vi "SolveContinousARE.vi"(8 "R":T3=[[1.0]], 9 "Q":T3=[[10.0, 0.0], [0.0, 100.0]], 10 "B":T3=[[0.0], [1.0]], 11 "A":T3=[[0.0, 1.0], [0.0, -1.0]]) -> (3 "A x B":T1=[[-1.6028844918025698e-15+0.0i, -100.90089284923441+0.0i], [-0.09910715076567198+0.0i, -1.0000000000000013+0.0i]])   [LabVIEW 2017]
uses:
  <vilib>/Analysis/Matrix/Datatypes/RealMatrix.ctl
  <vilib>/Analysis/Matrix/Datatypes/ComplexMatrix.ctl
  <vilib>/Analysis/7linalg.llb/Eigenvalue Order.ctl
  <vilib>/Analysis/baseanly.llb/Real A x B.vi
  <vilib>/Analysis/baseanly.llb/Complex A x B.vi
  <vilib>/Analysis/7linalg.llb/Complex Schur Decomposition.vi
  <vilib>/Analysis/baseanly.llb/Real Inverse Matrix.vi
  <vilib>/Analysis/Matrix/Numeric/Multiply/Multiply - CM,C.vi
  <vilib>/Analysis/Matrix/Numeric/Multiply/Multiply - RM,R.vi
  <vilib>/Analysis/baseanly.llb/Complex Inverse Matrix.vi
  <vilib>/Analysis/NI_AALBase.lvlib
  <vilib>/Analysis/Matrix/NI_Matrix.lvlib
  <vilib>/Analysis/NI_AALPro.lvlib
panel:
  out "Schur Form":T1=[[-0.3148128821469594+0.0i, -9.942271556684195+0.0i, 1.0334689231827774+0.0i, -0.5264552948285609+0.0i], [0.0+0.0i, 0.31481288214695996+0.0i, -1.133685179212674+0.0i, 10.823610418205856+0.0i], [0.0+0.0i, 0.0+0.0i, -10.044943645896394+0.0i, 98.40919793662512+0.0i], [0.0+0.0i, 0.0+0.0i, 0.0+0.0i, 10.044943645896401+0.0i]]
  in  "order":T2=3 items=["No Reorder", "Real Ascending", "Real Descending", "Magnitude Ascending", "Magnitude Descending"]
  in  "compute Schur vectors?":bool=TRUE
  out "Schur Vectors":T1=[[0.03146343137696174+0.0i, 0.9946277237284836+0.0i, -0.09801613012567584+0.0i, -0.010889532215374387+0.0i], [-0.00990509351401406+0.0i, 0.0003036415153823764+0.0i, -0.1105117271789722+0.0i, 0.9938254147888498+0.0i], [0.9994327793191794+0.0i, -0.03063770000817792+0.0i, 0.008706362771877389+0.0i, 0.010938473743360945+0.0i], [0.006786842476932152+0.0i, -0.09887836128665833+0.0i, -0.9889915043307461+0.0i, -0.1098763523241783+0.0i]]
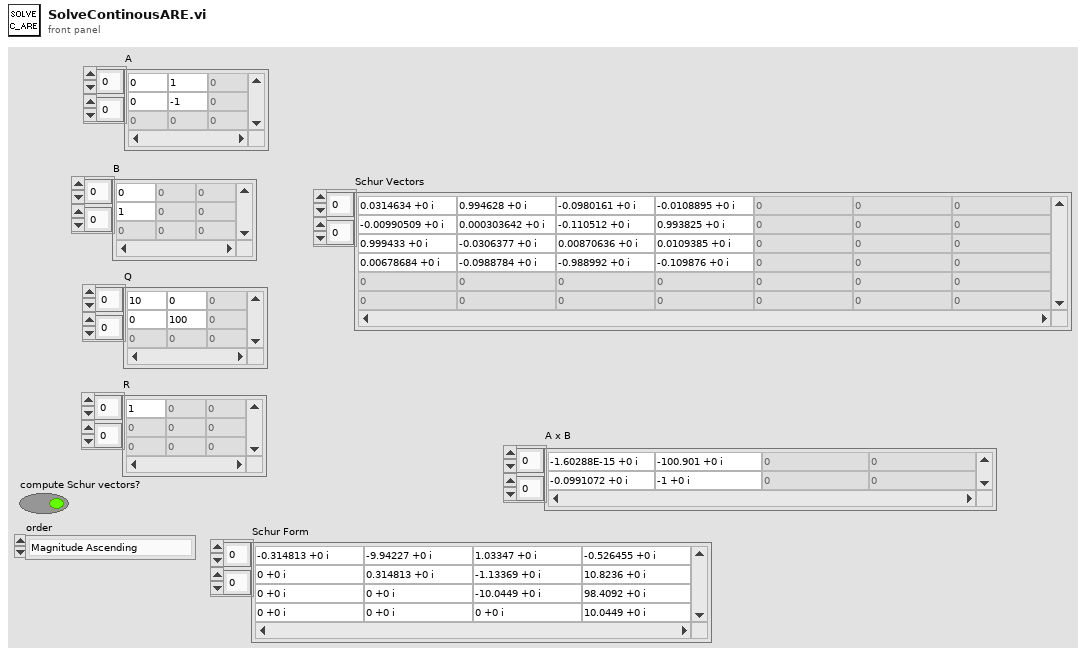
[diagram p1: front panel]
types:
  T1 = typedef "NI_Matrix.lvlib/ComplexMatrix.ctl" = cdb[][]
  T2 = typedef "NI_AALPro.lvlib/Eigenvalue Order.ctl" = u16
  T3 = typedef "NI_Matrix.lvlib/RealMatrix.ctl" = dbl[][]
  T4 = typedef "NI_Matrix.lvlib/RealMatrix.ctl" = cdb[][]
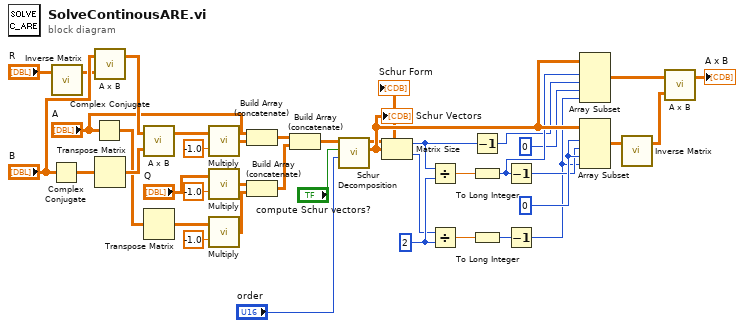
[diagram p0: block diagram]
diagram:
  w18 = 0 ("row 1")
  w17 = 2 ("y")
  n1 = Complex Conjugate(1:"B") -> (0:w39:T4)
  n2 = call-poly <vilib>:"Inverse Matrix.vi"("Input Matrix"="R") -> ("Inverse Matrix"=w35:T3)  [unwired: 1 in, 1 out]
  n3 = Complex Conjugate(1:"A") -> (0:w30:T4)
  n4 = call-poly <vilib>:"A x B.vi"("B"=w35, "A"="B") -> ("A x B"=w37:T3)  [unwired: 1 out]
  n5 = Transpose Matrix(1:w39) -> (0:w36:T4)
  n6 = call-poly <vilib>:"A x B.vi"("B"=w36, "A"=w37) -> ("A x B"=w32:T1)  [unwired: 1 out]
  n7 = Transpose Matrix(1:w30) -> (0:w28:T4)
  n8 = call-poly <vilib>:"Multiply.vi"("Complex Scalar c"=-1.0, "Complex Matrix A"=w32) -> ("A * c"=w26:T1)
  n9 = call-poly <vilib>:"Multiply.vi"("Real Scalar c"=-1.0, "Real Matrix A"="Q") -> ("A * c"=w25:T3)
  n10 = call-poly <vilib>:"Multiply.vi"("Complex Scalar c"=-1.0, "Complex Matrix A"=w28) -> ("A * c"=w24:T1)
  n11 = Build Array (concatenate)("A", w26) -> (w23:T1)
  n12 = Build Array (concatenate)(w25, w24) -> (w22:T1)
  n13 = Build Array (concatenate)(w23, w22) -> (w21:T1)
  n14 = call-poly <vilib>:"Schur Decomposition.vi"("order"="order", "compute Schur vectors?"="compute Schur vectors?", "Input Matrix"=w21) -> ("Schur Vectors"=w14:T1, "Schur Form"=→"Schur Form":T1)  [unwired: 5 in, 2 out]
  "Schur Vectors" <- w14
  n15 = Matrix Size(0:w14) -> (1:w7:i32, 2:w12:i32)
  n16 = Divide(x=w7, y=w17) -> (x/y=w16:dbl)
  n17 = Divide(x=w12, y=w17) -> (x/y=w15:dbl)
  n18 = Decrement(x=w7) -> (x-1=w6:i32)
  n19 = To Long Integer(number=w16) -> (32bit integer=w11:i32)
  n20 = To Long Integer(number=w15) -> (32bit integer=w10:i32)
  n21 = Decrement(x=w11) -> (x-1=w13:i32)
  n22 = Decrement(x=w10) -> (x-1=w8:i32)
  n23 = Array Subset(array=w14, index (row)=w11, length (row)=w6, index (col)=0 ("column 1"), length (col)=w8) -> (w4:T1)
  n24 = Array Subset(array=w14, index (row)=w18, length (row)=w13, index (col)=w18, length (col)=w8) -> (w5:T1)
  n25 = call-poly <vilib>:"Inverse Matrix.vi"("Input Matrix"=w5) -> ("Inverse Matrix"=w3:T1)  [unwired: 1 in, 1 out]
  n26 = call-poly <vilib>:"A x B.vi"("B"=w3, "A"=w4) -> ("A x B"=→"A x B":T1)  [unwired: 1 out]
